vi "Write With Abort.vi"(4 "size (unlimited)":i32, 6 "abort":bool, 7 "timeout in ms (-1)":i32=-1, 9 "last element? (F)":bool, 10 "element":T1, 11 "element valid? (T)":bool=TRUE) -> (1 "aborted?":bool, 2 "channel":T2, 3 "count":i32, 5 "timed out?":bool)   [LabVIEW 2017, in "Stream-t'WPI_EncoderType.ctl'.lvlib"]
doc: "Writes an element to a Stream channel or signals the channel to abort. The endpoint waits if the channel is full. This endpoint is the same as the Write endpoint except that it has an <B>abort</B> input and an <B>aborted?</B> output. You can use the abort capability of the Stream channel to close a channel abruptly, ignoring any data left in the channel buffer. You must use this endpoint together with the Read With Abort endpoint."
uses:
  <extravilib>/ChannelInstances/Stream-t'WPI_EncoderType.ctl'.lvlib
  <extravilib>/ChannelInstances/Stream-t'WPI_EncoderType.ctl'/)Channel.ctl
  <vilib>/Rock Robotics/WPI/Encoder/WPI_EncoderType.ctl
  <resource>/ChannelSupport/_ChannelSupport/WaitIfNeeded.vi
  <extravilib>/ChannelInstances/Stream-t'WPI_EncoderType.ctl'/)Channel.vi
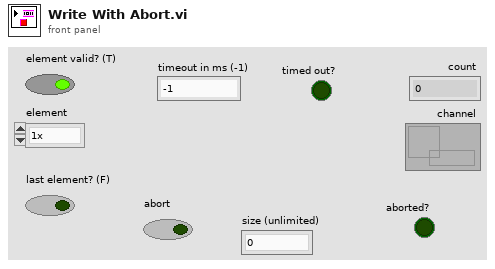
[diagram p1: front panel]
types:
  T1 = typedef "WPI_EncoderType.ctl" = enum16{"1x", "2x", "4x"}
  T2 = typedef "Stream-t'WPI_EncoderType.ctl'.lvlib/)Channel.ctl" = refnum<queue>
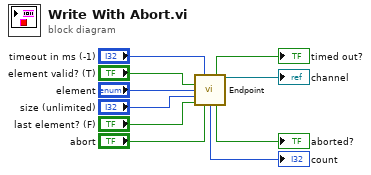
[diagram p0: block diagram]
diagram:
  n1 = call <extravilib>:"Endpoint.vi"("timeout in ms (-1)"="timeout in ms (-1)", "is valid (T)"="element valid? (T)", "element in"="element", "size (0)"="size (unlimited)", "is last element (F)"="last element? (F)", "abort (F)"="abort") -> ("timed out?"=→"timed out?":bool, "channel out"=→"channel":T2, "count"=→"count":i32, "aborted?"=→"aborted?":bool)  [unwired: 6 in]
